vi "Database.StatusUpdate.vi"(8 "error in (no error)":errorcluster, 11 "Data in":T1) -> (0 "error out":errorcluster, 3 "Data out":T1)   [LabVIEW 2016]
uses:
  Database.Data.ctl
  Database.Data.Sets.ctl
  Handler/Database.Handler.Data.Status.ctl
  Database.Global.vi
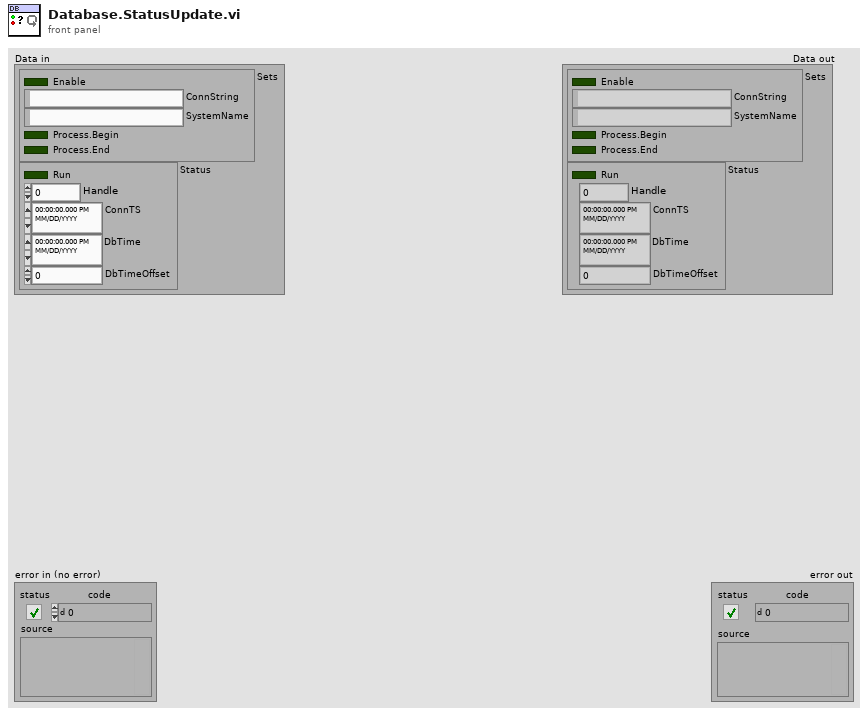
[diagram p1: front panel]
types:
  T1 = typedef "Database.Data.ctl" = cluster{"Sets":T2, "Status":T3}
  T2 = typedef "Database.Data.Sets.ctl" = cluster{"Enable":bool, "ConnString":string, "SystemName":string, "Process.Begin":bool, "Process.End":bool}
  T3 = typedef "Database.Handler.Data.Status.ctl" = cluster{"Run":bool, "Handle":i32, "ConnTS":timestamp, "DbTime":timestamp, "DbTimeOffset":dbl}
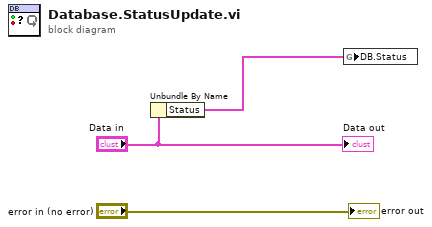
[diagram p0: block diagram]
diagram:
  n1 = Unbundle By Name("Data in") -> ("Status"=w1:T3)
  n2 = global write "Database.Global.vi" "DB.Status"(w1) -> ()
  "Data out" <- "Data in"
  "error out" <- "error in (no error)"
